vi "设置二维数组值.vi"(1 "数值":i32, 2 "索引":i32, 3 "数组":i32[][](array[numeric])) -> (0 "输出数组":i32[][](array[numeric]))   [LabVIEW 2017]
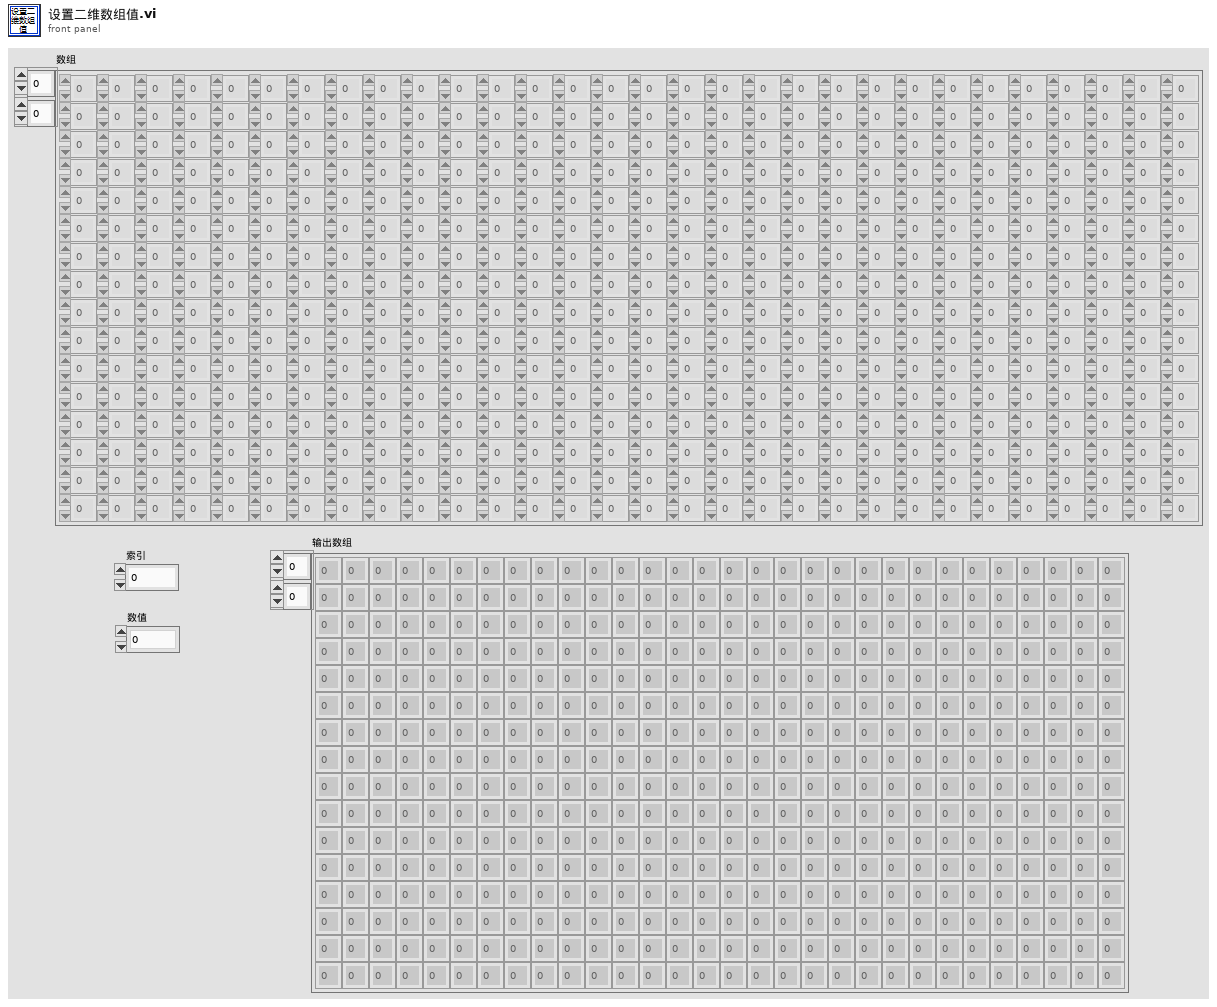
[diagram p1: front panel]
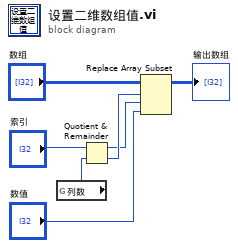
[diagram p0: block diagram]
diagram:
  n1 = global read "全局变量.vi" "列数"() -> (w1:i32)
  n2 = Quotient & Remainder(x="索引", y=w1) -> (x-y*floor(x/y)=w3:i32, floor(x/y)=w4:i32)
  n3 = Replace Array Subset(array="数组", new element="数值", index (row)=w4, index (col)=w3) -> (→"输出数组":i32[][])
